vi "mjpegReader.vi"() -> ()   [LabVIEW 2024]
uses:
  System.Drawing
panel:
  out "Image":T1(plugin-control)
  in  "Footer":i32=2
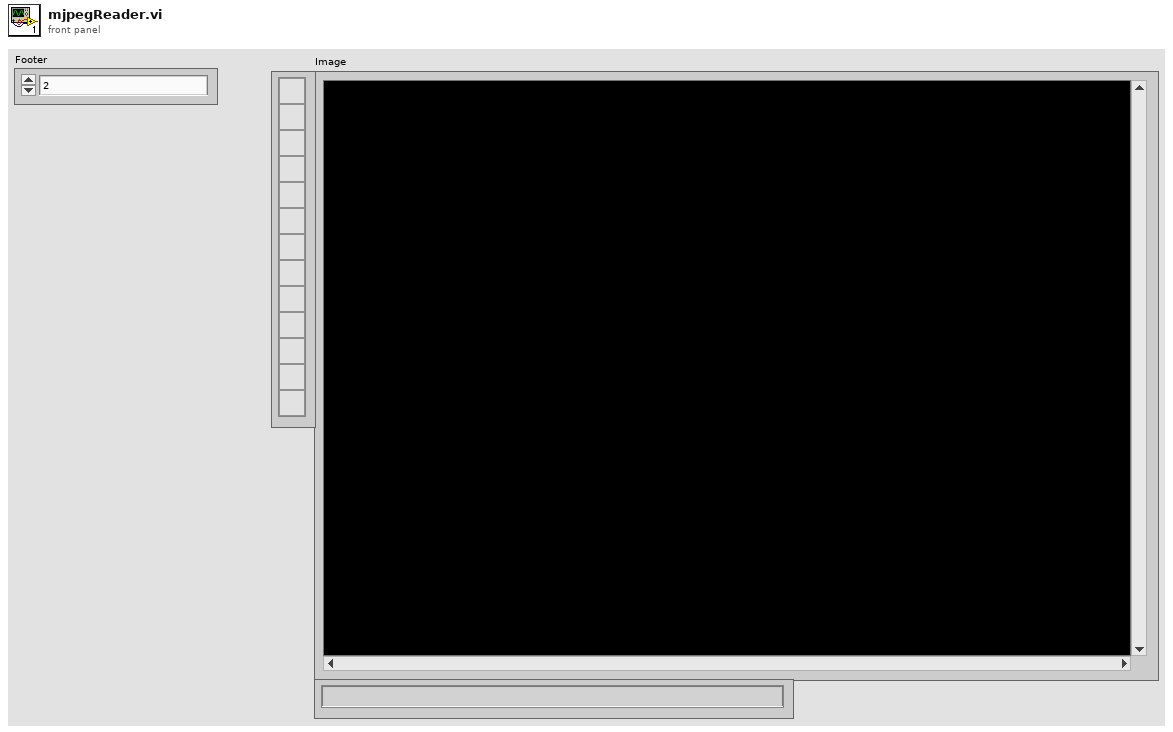
[diagram p1: front panel]
types:
  T1 = typedef "IMAQ Image.ctl" = refnum<image>
  T2 = typedef "Image Type" = u32
  T3 = typedef "imagedata.ctl" = cluster{"image type":i32, "image depth":i32, "image":u8[], "mask":u8[], "colors":u32[], "Rectangle":cluster{"left":i16, "top":i16, "right":i16, "bottom":i16}}
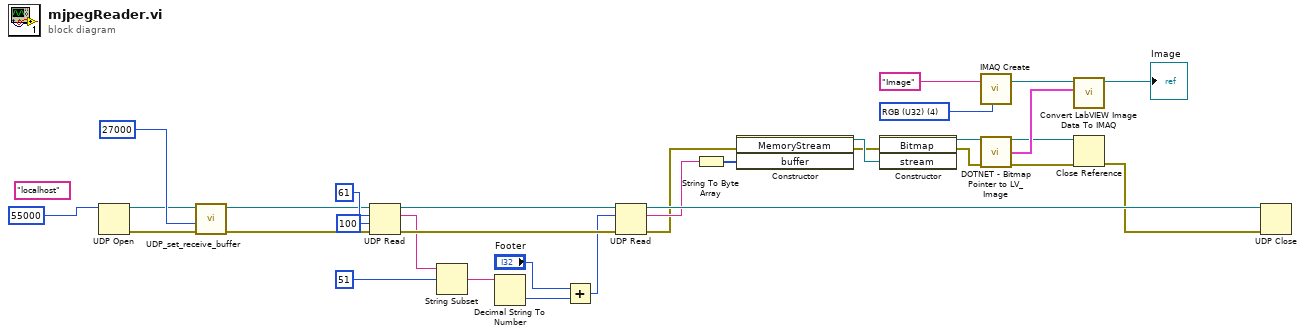
[diagram p0: block diagram]
diagram:
  (unwired) "localhost" ("address")
  w15 = T2 4 items=["Grayscale (U8)", "Grayscale (I16)", "Grayscale (SGL)", "Complex (CSG)", "RGB (U32)", "HSL (U32)", "RGB (U64)", "Grayscale (U16)"] ("Image Type")
  n1 = UDP Open(11:u16 55000 ("remote port or service name")) -> (port=w2:refnum<k16>, 0:w4:errorcluster)  [unwired: 4 in, 1 out]
  n2 = call "UDP_set_receive_buffer.vi"("error in (no error)"=w4, "Receive Buffer Size"=u32 27000, "connection ID"=w2) -> ("error out"=w3:errorcluster, "connection ID out"=w1:refnum<k16>)  [unwired: 6 in]
  n3 = UDP Read(connection ID=w1, max size (548)=61 ("bytes to read"), timeout ms (25000)=100, 8:w3) -> (data out=w23:string, error out=w30:errorcluster, 3:w29:refnum<k16>)  [unwired: 2 out]
  n4 = String Subset(string=w23, offset (0)=51) -> (substring=w22:string)  [unwired: 1 in]
  n5 = Decimal String To Number(string=w22) -> (number=w19:i32)  [unwired: 2 in, 1 out]
  n6 = Add(x="Footer", y=w19) -> (x+y=w18:i32)
  n7 = UDP Read(connection ID=w29, max size (548)=w18, 8:w30) -> (data out=w24:string, error out=w9:errorcluster, 3:w32:refnum<k16>)  [unwired: 1 in, 2 out]
  n8 = String To Byte Array(string=w24) -> (unsigned byte array=w25:u8[])
  n9 = constructor class="MemoryStream"(error in=w9, "buffer"=w25) -> (reference out=w28:refnum<k24>, error out=w26:errorcluster)  [unwired: 2 in, 2 out]
  n10 = constructor class="Bitmap"(error in=w26, "stream"=w28) -> (reference out=w11:refnum<k24>, error out=w27:errorcluster)  [unwired: 2 in, 2 out]
  n11 = call "IMAQ Create"("Image Name"="Image", "Image Type"=w15) -> ("New Image"=w13:T1)  [unwired: 3 in, 1 out]
  n12 = call "DOTNET - Bitmap Pointer to LV_Image.vi"("Bitmap"=w11, "error in (no error)"=w27) -> ("Bitmap dup"=w8:refnum<k24>, "LV_Image"=w16:T3, "error out"=w10:errorcluster)  [unwired: 10 in, 1 out]
  n13 = call "Convert LabVIEW Image Data To IMAQ.vi"("Image Data"=w16, "Image In"=w13) -> ("Image Out"=→"Image":T1)  [unwired: 8 in, 1 out]
  n14 = Close Reference(reference=w8, error in (no error)=w10) -> (error out=w31:errorcluster)
  n15 = UDP Close(connection ID=w32, 8:w31) -> ()  [unwired: 2 out]
